vi "createYi_.vi"(9 "Min":dbl, 10 "Max":dbl, 11 "delta":dbl) -> (2 "max value":dbl, 3 "Array":dbl[](array[numeric]))   [LabVIEW 2020]
uses:
  NI_AALBase.lvlib
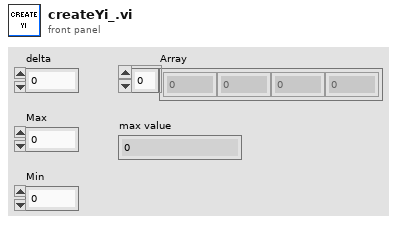
[diagram p1: front panel]
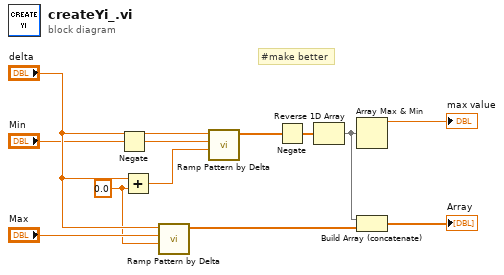
[diagram p0: block diagram]
diagram:
  w5 = 0.0 ("start")
  # "#make better"
  n1 = Negate(x="Min") -> (-x=w6:dbl)
  n2 = Add(x="delta", y=w5) -> (x+y=w4:dbl)
  n3 = call "Ramp Pattern by Delta.vi"("start"=w5, "end"="Max", "delta"="delta") -> ("Ramp Pattern"=w8:dbl[])  [unwired: 6 in, 2 out]
  n4 = call "Ramp Pattern by Delta.vi"("start"=w4, "end"=w6, "delta"="delta") -> ("Ramp Pattern"=w3:dbl[])  [unwired: 6 in, 2 out]
  n5 = Negate(x=w3) -> (-x=w2:dbl[])
  n6 = Reverse 1D Array(array=w2) -> (reversed array=w1:dbl[])
  n7 = Array Max & Min(array=w1) -> (max value=→"max value":dbl)  [unwired: 3 out]
  n8 = Build Array (concatenate)(w1, w8) -> (→"Array":dbl[])
